vi "Import - UDP Custom Device.vi"(6 "New CD?":bool, 8 "error in (no error)":errorcluster, 10 "Target File":path, 11 "Device Item Ref in":T1 format="%.0x") -> (0 "error out":errorcluster)   [LabVIEW 2019, in "UDP-Custom-Device System Explorer.lvlib"]
uses:
  UDP-Custom-Device System Explorer.lvlib
  <vilib>/NI VeriStand/Custom Device API/Custom Device Item Ref.ctl
  <vilib>/NI VeriStand/Custom Device API/Custom Device API.lvlib
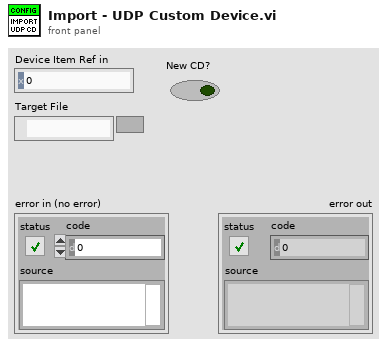
[diagram p1: front panel]
types:
  T1 = typedef "Custom Device API.lvlib/Custom Device Item Ref.ctl" = u64
  T2 = typedef "UDP-Custom-Device System Explorer.lvlib/ImpExp - Data.ctl" = cluster{"Import/Export Data - Main":T3, "Rx Packets":T5, "Tx Packets":T14}
  T3 = typedef "UDP-Custom-Device System Explorer.lvlib/ImpExp - Main Data.ctl" = cluster{"Common":T4, "Export File Location":path, "Export to File Status":bool, "Timestamp Path":string, "Description":string}
  T4 = typedef "Custom Device API.lvlib/Custom Device Item Info.ctl" = cluster{"Name":string, "Is Channel":bool, "GUID":string, "Is Waveform":bool}
  T5 = typedef "UDP-Custom-Device System Explorer.lvlib/ImpExp - Rx Packets Data.ctl" = cluster{"Common":T4, "Packet Names":string[], "Packet IDs":i32[], "Packet Paths":string[], "Rx Packet Data":T6[]}
  T6 = typedef "UDP-Custom-Device System Explorer.lvlib/ImpExp - Rx Packet Data.ctl" = cluster{"Common":T4, "Packet ID":i32, "Header Info":u32, "Auto-Assign NIC":bool, "IP Address of Local NIC":string, "Port":u16, "Read Timeout":i32, "Endianness":u16, "Channel Names":string[], "Data Types":T7[], "Description":string, "Buffered Packet Info":T8, "Multicast IP":string, "Multicast?":bool, "New Data Option":T12, "Debug Mode":bool, "targetProcessor":i8, "targetPriority":i16, "Thread Mgmt":T13}
  T7 = typedef "UDP-Custom-Device Shared.lvlib/Shared - Channel Data Type.ctl" = enum16{"Boolean", "Single", "Double", "I8", "I16", "I32", "I64", "U8", "U16", "U32", "U64"}
  T8 = typedef "UDP-Custom-Device Shared.lvlib/Shared - Buffered.PacketInfo.ctl" = cluster{"Buffer Size":i32, "External Buffer":bool, "Prepend Header":bool, "Is Buffered":bool, "Pointer Encoding":T9, "Rx Buffer Option":T10, "Tx Buffer Option":T11}
  T9 = typedef "UDP-Custom-Device Shared.lvlib/Shared - Pointer Encoding.ctl" = enum16{"Direct Encoding", "Conversion Encoding"}
  T10 = typedef "UDP-Custom-Device Shared.lvlib/Shared - Receive Buffer Options.ctl" = enum16{"Static Buffer", "Circular Buffer", "Circular Buffer + Size", "Internal Cache", "Internal Cache + Size", "Ping Pong", "Ping Pong + Size"}
  T11 = typedef "UDP-Custom-Device Shared.lvlib/Shared - Transmit Buffer Options.ctl" = enum16{"Static Buffer", "FIFO Buffer", "FIFO Buffer + Port"}
  T12 = typedef "UDP-Custom-Device Shared.lvlib/Shared - New Data Options.ctl" = enum16{"Timeout Reset", "Counter"}
  T13 = typedef "UDP-Custom-Device Shared.lvlib/Shared - Thread Management.ctl" = enum16{"Untimed (Default)", "Timed (High Priority)"}
  T14 = typedef "UDP-Custom-Device System Explorer.lvlib/ImpExp - Tx Packets Data.ctl" = cluster{"Common":T4, "Packet IDs":i32[], "Packet Names":string[], "Packet Paths":string[], "Tx Packet Data":T15[]}
  T15 = typedef "UDP-Custom-Device System Explorer.lvlib/ImpExp - Tx Packet Data.ctl" = cluster{"Common":T4, "Packet ID":i32, "Header Info":u32, "Auto-Assign NIC":bool, "IP Address of Local NIC":string, "Port":u16, "Destination IP":string, "Destination Port":u16, "Endianness":u16, "Channel Names":string[], "Channel Paths":string[], "Data Types":T7[], "Timestamp Path":string, "Description":string, "Buffered Packet Info":T8, "Multicast IP":string, "Multicast?":bool, "TTL":u16, "Port as Channel?":bool, "Transmit Option":T16, "Transmit Echo Option":T17, "Debug Mode":bool, "threadOptions":T18}
  T16 = typedef "UDP-Custom-Device Shared.lvlib/Shared - Transmit Flag Options.ctl" = enum16{"Always", "One-Shot", "Toggle"}
  T17 = typedef "UDP-Custom-Device Shared.lvlib/Shared - Transmit Echo Options.ctl" = enum16{"PCL Reset", "Counter", "Mirror"}
  T18 = typedef "UDP-Custom-Device System Explorer.lvlib/Thread Configuration.ctl" = cluster{"targetProcessor":i8, "targetPriority":i16, "Synchronization":T19, "loopPeriod":u32, "pclDecimation":u16, "threadManagement":T13}
  T19 = typedef "UDP-Custom-Device System Explorer.lvlib/Thread Sync Reference.ctl" = enum16{"PCL", "Async"}
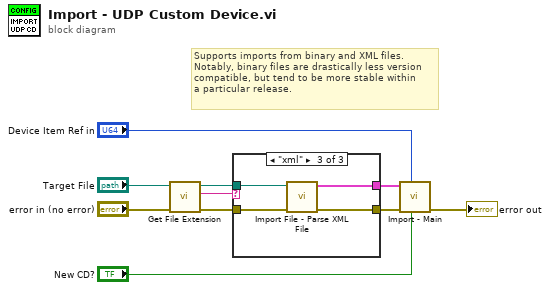
[diagram p0: block diagram]
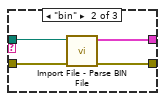
[diagram p3: hidden frame]
diagram:
  # "Supports imports from binary and XML files.\nNotably, binary files are drastically less version\ncompatible, but tend to be more stable within\na particular release."
  n1 = call <vilib>:"Get File Extension.vi"("error in (no error)"="error in (no error)", "file"="Target File") -> ("error out"=w2:errorcluster, "lowercase file extension"=w1:string, "dup file"=w4:path)  [unwired: 5 in, 2 out]
  n2 = case shown="\"xml\"" w1 {
    tunnel: [w11 w15 w16] -> w9
    tunnel: [_ w14 w18] -> w7
    tunnel: w4 -> [_ w13 w19]
    tunnel: w2 -> [w11 w12 w17]
    frame Default {
    }
    frame "bin" {
      n3 = call "Import File - Parse BIN File.vi"("error in (no error)"=w12, "Target File"=w13) -> ("error out"=w15:errorcluster, "Import/Export Data"=w14:T2)  [unwired: 8 in]
    }
    frame "xml" {
      n4 = call "Import File - Parse XML File.vi"("error in (no error)"=w17, "Target File"=w19) -> ("error out"=w16:errorcluster, "Import/Export Data"=w18:T2)  [unwired: 8 in]
    }
  }
  n5 = call "Import - Main.vi"("New CD?"="New CD?", "Device Item Ref in"="Device Item Ref in", "error in (no error)"=w9, "Import/Export Data"=w7) -> ("error out"=→"error out":errorcluster)  [unwired: 7 in]
